vi "CreatePersonnel.vi"(8 "error in (no error)":errorcluster, 9 "Role":T1, 10 "UniqueID":string, 11 "Name":string) -> (0 "error out":errorcluster, 3 "output cluster":refnum<class "Personnel.lvclass">)   [LabVIEW 2015, in "Personnel.lvclass"]
uses:
  Personnel.lvclass
  PersonnelType.ctl
  Personnel.lvclass/Personnel.ctl
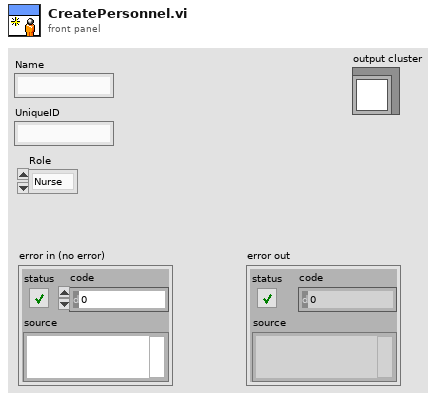
[diagram p1: front panel]
types:
  T1 = typedef "Personnel.lvclass/PersonnelType.ctl" = enum16{"Nurse", "Doctor", "Cleanning", "Admin"}
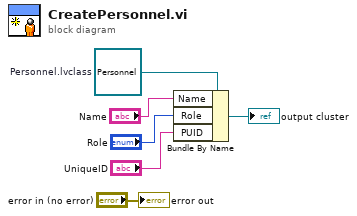
[diagram p0: block diagram]
diagram:
  w6 = refnum<class "Personnel.lvclass"> refnum  # Personnel.lvclass
  n1 = Bundle By Name(cluster=w6, "Name"="Name", "Role"="Role", "PUID"="UniqueID") -> (→"output cluster":refnum<class "Personnel.lvclass">)
  "error out" <- "error in (no error)"
